vi "Children Allowed.vi"(8 "error in (no error)":errorcluster, 11 "BetterTreeItem in":refnum<class "Valve Item.lvclass">) -> (0 "error out":errorcluster, 2 "Child allowed?":bool, 3 "BetterTreeItem out":refnum<class "Valve Item.lvclass">)   [LabVIEW 2020, in "BetterDragAndDropDemo.lvlib" / "Valve Item.lvclass"]
uses:
  Valve Item.lvclass
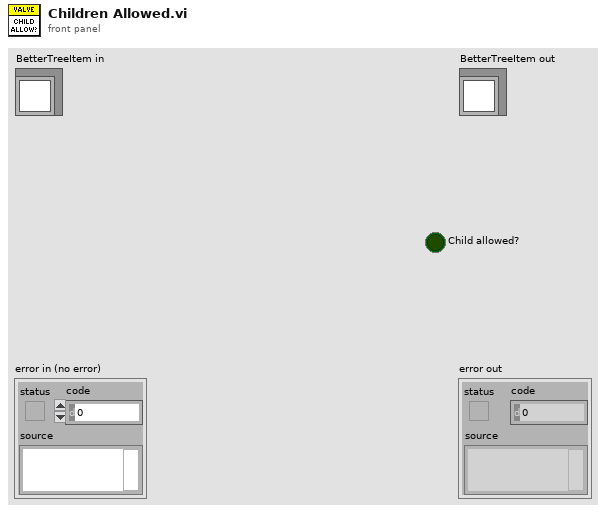
[diagram p1: front panel]
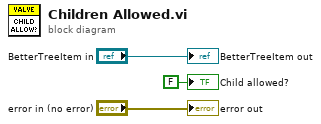
[diagram p0: block diagram]
diagram:
  "error out" <- "error in (no error)"
  "BetterTreeItem out" <- "BetterTreeItem in"
  "Child allowed?" <- FALSE ("Child allowed?")
